vi "Folder_SPCImporter_CWB.vi"() -> ()   [LabVIEW 2014]
uses:
  <vilib>/Utility/file.llb/Write To Spreadsheet File (string).vi
panel:
  out "SPECTRA":cluster{i32[], i32[]}[](graph)
  in  "Select folder with  .spc files to convert to one .csv file that contains the Raman data and one .csv file that contains to instrument information.":path=path "" caption="start path"
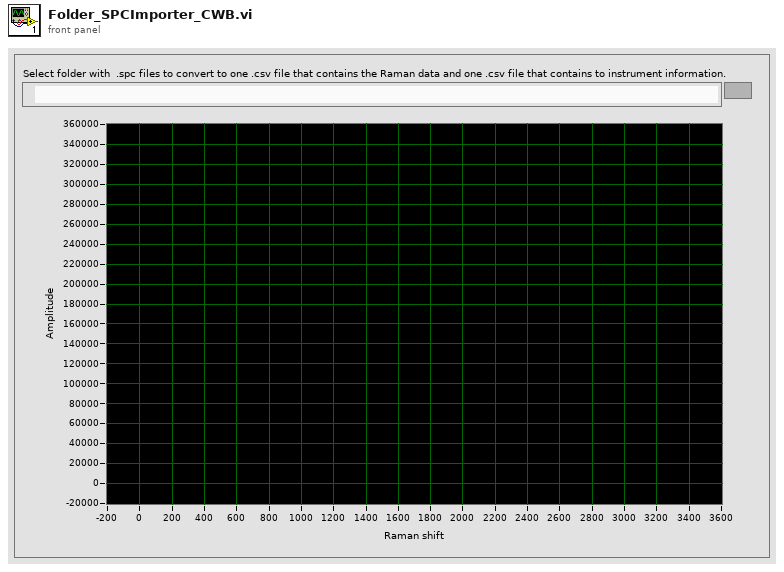
[diagram p1: front panel]
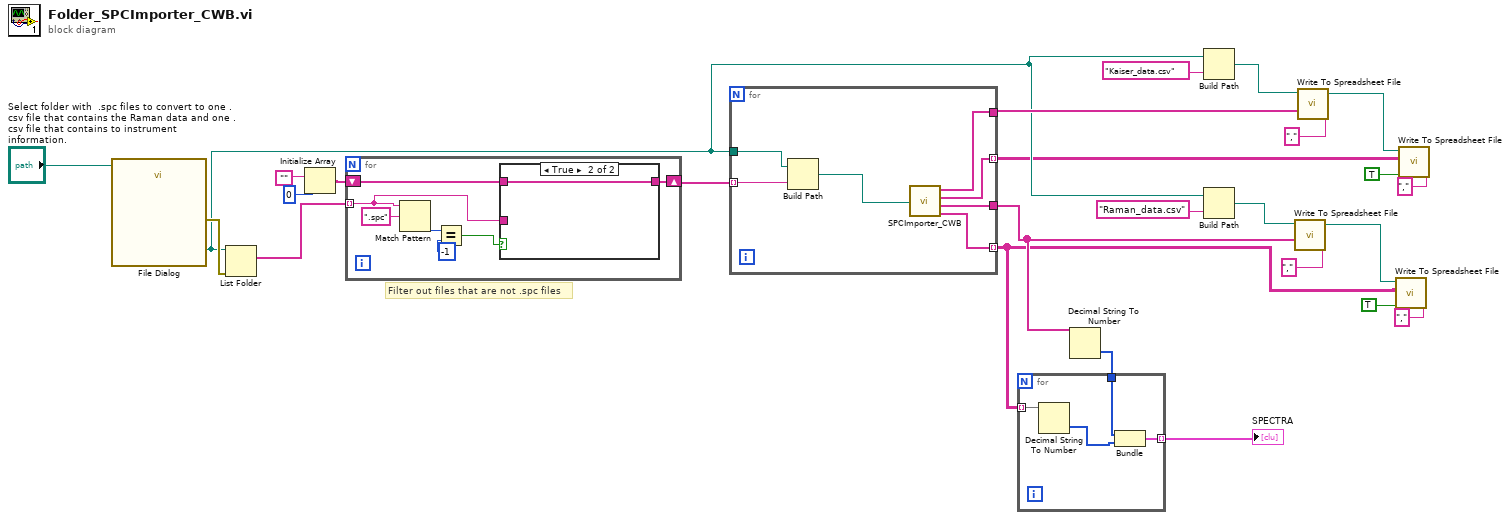
[diagram p0: block diagram]
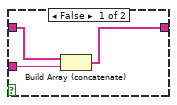
[diagram p2: hidden frame]
diagram:
  # "Filter out files that are not .spc files"
  n1 = call "File Dialog"("start path"="Select folder with  .spc files to convert to one .csv file that contains the Raman data and one .csv file that contains to instrument information.") -> ("selected path"=w7:path, "error out"=w26:errorcluster)  [unwired: 11 in, 2 out]
  n2 = List Folder(path=w7, error in=w26) -> (filenames=w22:string[])  [unwired: 2 in, 3 out]
  n3 = Initialize Array("", 0 ("dimension size")) -> (w25:string[])
  n4 = for {
    tunnel: w22 -> [w29] mode=indexing
    shift-right: [w27] -> w21
    shift-left: w25 -> [w28]
    n5 = Match Pattern(string=w29, regular expression=".spc") -> (offset past match=w32:i32)  [unwired: 1 in, 3 out]
    n6 = Equal?(x=w32, y=-1) -> (x = y?=w30:bool)
    n7 = case shown="True" w30 {
      tunnel: w29 -> [w36 _]
      tunnel: w28 -> [w35 w37]
      tunnel: [w34 w37] -> w27
      frame False {
        n8 = Build Array (concatenate)(w35, w36) -> (w34:string[])
      }
      frame True {
      }
    }
  }
  n9 = for {
    tunnel: w7 -> [w44]
    tunnel: w21 -> [w43] mode=indexing
    tunnel: [w41] -> w8
    tunnel: [w40] -> w6 mode=indexing
    tunnel: [w39] -> w4
    tunnel: [w38] -> w3 mode=indexing
    n10 = Build Path(base path=w44, name or relative path=w43) -> (appended path=w42:path)
    n11 = call "SPCImporter_CWB.vi"("start path"=w42) -> ("Kaiser labels"=w41:string[], "Kaiser data"=w40:string[], "Raman labels"=w39:string[], "Raman data"=w38:string[])
  }
  n12 = Decimal String To Number(string=w4) -> (number=w2:i32[])  [unwired: 2 in, 1 out]
  n13 = for {
    tunnel: w3 -> [w48] mode=indexing
    tunnel: w2 -> [w46]
    tunnel: [w45] -> w1 mode=indexing
    n14 = Decimal String To Number(string=w48) -> (number=w47:i32[])  [unwired: 2 in, 1 out]
    n15 = Bundle(w46, w47) -> (w45:cluster{i32[], i32[]})  [unwired: 1 in]
  }
  "SPECTRA" <- w1
  n16 = Build Path(base path=w7, name or relative path="Kaiser_data.csv") -> (appended path=w9:path)
  n17 = Build Path(base path=w7, name or relative path="Raman_data.csv") -> (appended path=w14:path)
  n18 = call-poly <vilib>:"Write To Spreadsheet File.vi"("delimiter (\\t)"="," ("delimiter (\\t)"), "1D data"=w4, "file path (dialog if empty)"=w14) -> ("new file path (Not A Path if cancelled)"=w15:path)  [unwired: 5 in]
  n19 = call-poly <vilib>:"Write To Spreadsheet File.vi"("delimiter (\\t)"="," ("delimiter (\\t)"), "1D data"=w8, "file path (dialog if empty)"=w9) -> ("new file path (Not A Path if cancelled)"=w10:path)  [unwired: 5 in]
  n20 = call-poly <vilib>:"Write To Spreadsheet File.vi"("delimiter (\\t)"="," ("delimiter (\\t)"), "append to file? (new file:F)"=TRUE, "2D data"=w3, "file path (dialog if empty)"=w15) -> ()  [unwired: 4 in, 1 out]
  n21 = call-poly <vilib>:"Write To Spreadsheet File.vi"("delimiter (\\t)"="," ("delimiter (\\t)"), "append to file? (new file:F)"=TRUE, "2D data"=w6, "file path (dialog if empty)"=w10) -> ()  [unwired: 4 in, 1 out]
